vi "Jeffress_model_v009.vi"() -> ()   [LabVIEW 2019]
panel:
  out "element 2":dbl
  out "Elapsed time 2":dbl caption="Get Start Time (s)"
  out "new picture":picture
  out "Left - Right":dbl
  out "Elapsed time 1":dbl caption="Get Start Time (s)"
  in  "stop":bool
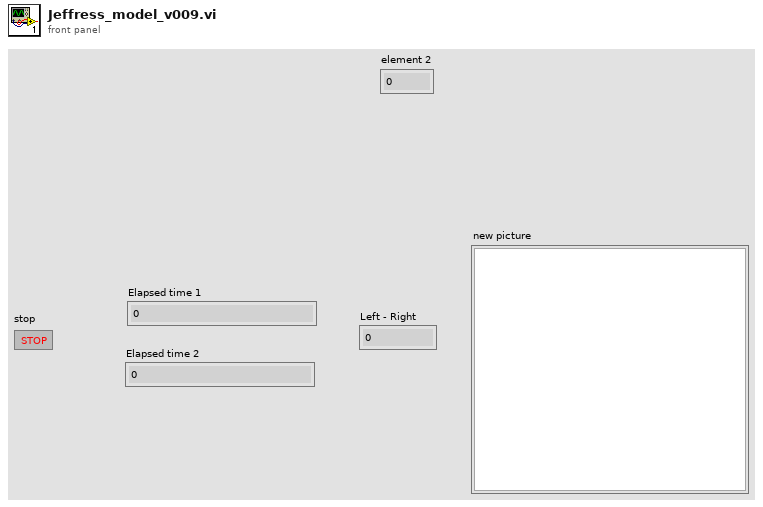
[diagram p1: front panel]
types:
  T1 = cluster{"maximum":dbl, "minimum":dbl, "clip to min":bool, "log?(F)":bool, "grid color":u32, "plot color":u32, "fmt and prec":cluster{"format":enum8{"Decimal", "Scientific", "Engineering", "Binary", "Octal", "Hex"}, "precision":u8}, "visible section":u16}
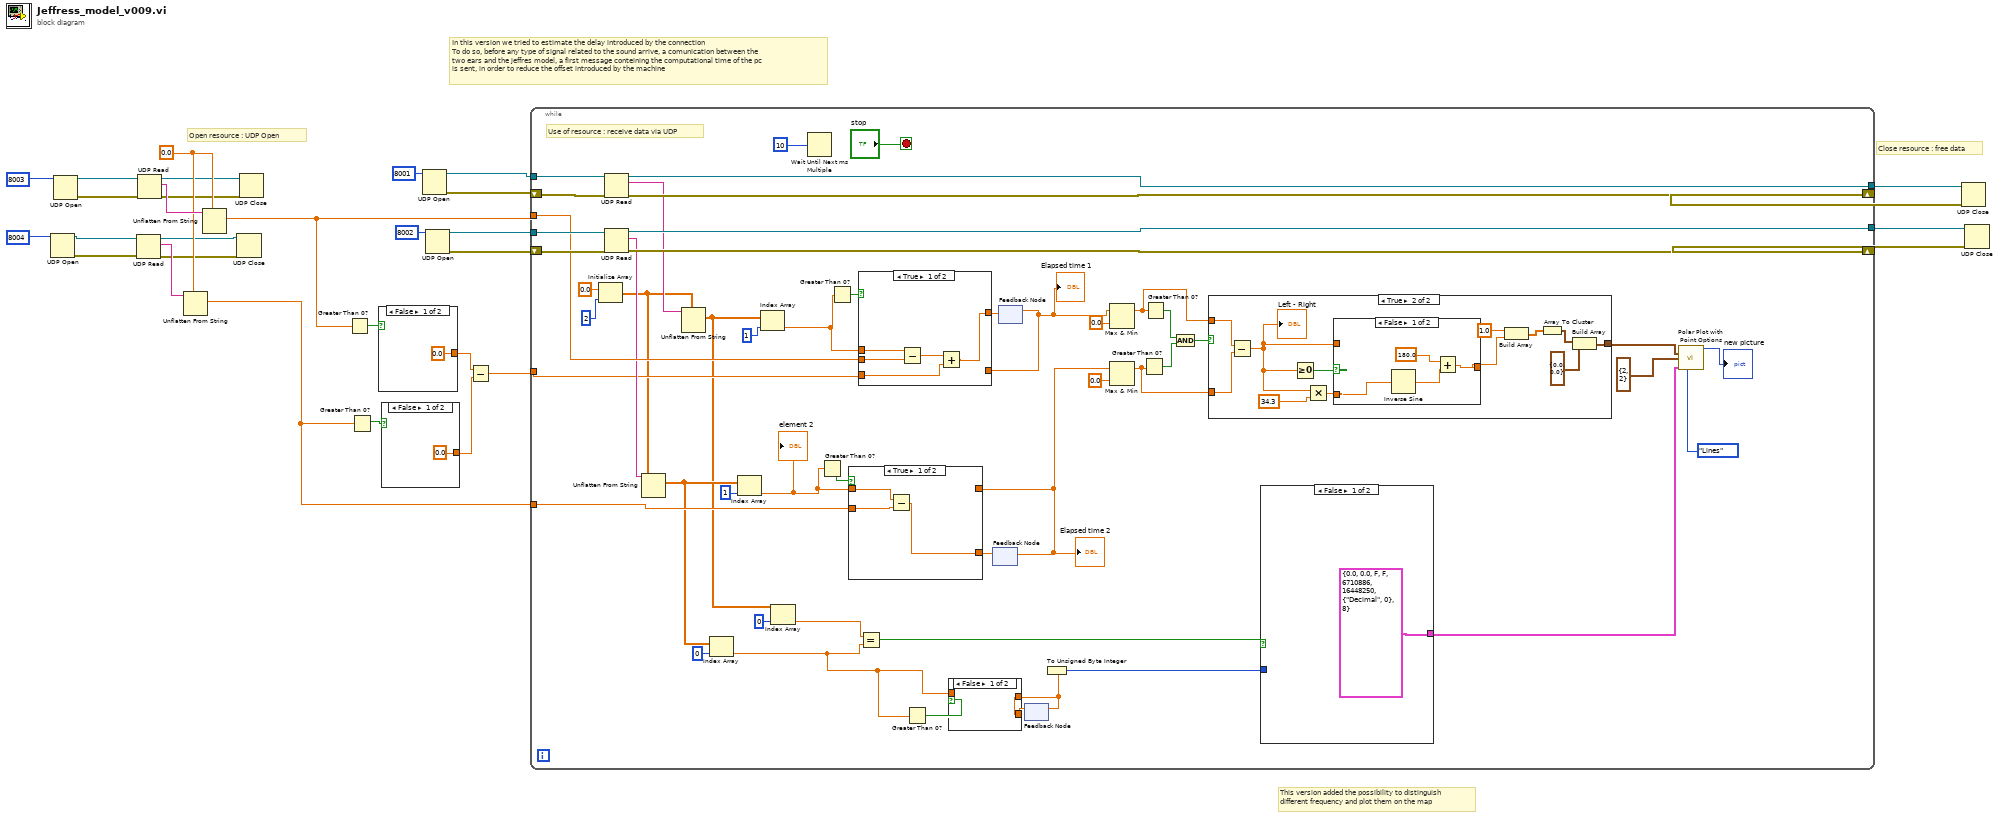
[diagram p0: block diagram]
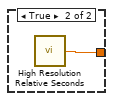
[diagram p2: hidden frame]
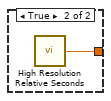
[diagram p3: hidden frame]
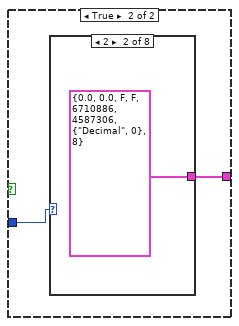
[diagram p5: hidden frame]
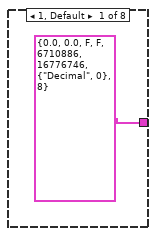
[diagram p6: hidden frame]
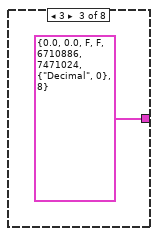
[diagram p7: hidden frame]
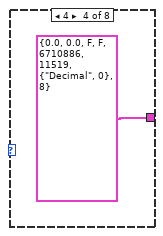
[diagram p8: hidden frame]
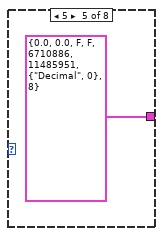
[diagram p9: hidden frame]
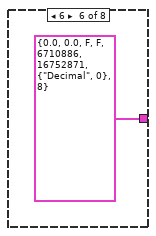
[diagram p10: hidden frame]
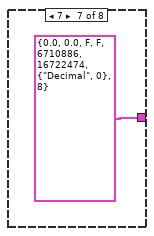
[diagram p11: hidden frame]
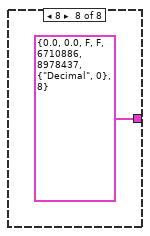
[diagram p12: hidden frame]
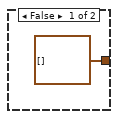
[diagram p14: hidden frame]
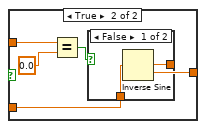
[diagram p15: hidden frame]
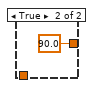
[diagram p16: hidden frame]
diagram:
  w18 = 0.0
  # "This version added the possibility to distinguish\ndifferent frequency and plot them on the map"
  # "In this version we tried to estimate the delay introduced by the connection\nTo do so, before any type of signal related to the sound arrive, a comunication between the\ntwo ears and the jeffres model, a first message conteining the computational time of the pc\nis sent, in order to reduce the offset introduced by the machine"
  # "Close resource : free data"
  # "Open resource : UDP Open"
  n1 = UDP Open(11:u16 8004) -> (port=w22:refnum<k16>, 0:w21:errorcluster)  [unwired: 4 in, 1 out]
  n2 = UDP Open(11:u16 8003) -> (port=w24:refnum<k16>, 0:w23:errorcluster)  [unwired: 4 in, 1 out]
  n3 = UDP Read(connection ID=w22, 8:w21) -> (data out=w19:string, error out=w14:errorcluster, 3:w15:refnum<k16>)  [unwired: 2 in, 2 out]
  n4 = UDP Read(connection ID=w24, 8:w23) -> (data out=w20:string, error out=w16:errorcluster, 3:w17:refnum<k16>)  [unwired: 2 in, 2 out]
  n5 = Unflatten From String(type=w18, binary string=w19) -> (value=w4:dbl)  [unwired: 3 in, 2 out]
  n6 = Unflatten From String(type=w18, binary string=w20) -> (value=w6:dbl)  [unwired: 3 in, 2 out]
  n7 = UDP Close(connection ID=w15, 8:w14) -> ()  [unwired: 2 out]
  n8 = UDP Close(connection ID=w17, 8:w16) -> ()  [unwired: 2 out]
  n9 = Greater Than 0?(x=w6) -> (x > 0?=w7:bool)
  n10 = Greater Than 0?(x=w4) -> (x > 0?=w5:bool)
  n11 = case shown="False" w7 {
    tunnel: [0.0 ("relative seconds") w32] -> w3
    frame False {
    }
    frame True {
      n12 = call <vilib>:"High Resolution Relative Seconds.vi"() -> ("relative seconds"=w32:dbl)
    }
  }
  n13 = case shown="False" w5 {
    tunnel: [0.0 ("relative seconds") w34] -> w2
    frame False {
    }
    frame True {
      n14 = call <vilib>:"High Resolution Relative Seconds.vi"() -> ("relative seconds"=w34:dbl)
    }
  }
  n15 = UDP Open(11:u16 8001 ("port")) -> (port=w13:refnum<k16>, 0:w12:errorcluster)  [unwired: 4 in, 1 out]
  n16 = UDP Open(11:u16 8002 ("port")) -> (port=w11:refnum<k16>, 0:w10:errorcluster)  [unwired: 4 in, 1 out]
  n17 = Subtract(x=w3, y=w2) -> (x-y=w1:dbl)
  n18 = while {
    tunnel: w13 -> [w81]
    tunnel: [w80] -> w29
    shift-right: [w83] -> w30
    shift-left: w12 -> [w82]
    tunnel: w11 -> [w69]
    tunnel: [w67] -> w25
    shift-right: [w68] -> w26
    shift-left: w10 -> [w66]
    tunnel: w4 -> [w59]
    tunnel: w6 -> [w58]
    tunnel: w1 -> [w54]
    stop <- "stop" stop-if-true
    # "Use of resource : receive data via UDP"
    n19 = Initialize Array(0.0 ("element"), 2 ("dimension size")) -> (w51:dbl[])
    n20 = UDP Read(connection ID=w81, 8:w82) -> (data out=w61:string, error out=w83:errorcluster, 3:w80:refnum<k16>)  [unwired: 2 in, 2 out]
    n21 = UDP Read(connection ID=w69, 8:w66) -> (data out=w56:string, error out=w68:errorcluster, 3:w67:refnum<k16>)  [unwired: 2 in, 2 out]
    n22 = Unflatten From String(type=w51, binary string=w56) -> (value=w47:dbl[])  [unwired: 3 in, 2 out]
    n23 = Unflatten From String(type=w51, binary string=w61) -> (value=w46:dbl[])  [unwired: 3 in, 2 out]
    n24 = Index Array(array=w47, index=0) -> (element=w37:dbl)
    n25 = Index Array(array=w47, index=1) -> (element=w41:dbl)
    "element 2" <- w41
    n26 = Index Array(array=w46, index=1) -> (element=w49:dbl)
    n27 = Index Array(array=w46, index=0) -> (element=w43:dbl)
    n28 = Wait Until Next ms Multiple(millisecond multiple=u32 10) -> ()  [unwired: 1 out]
    n29 = Greater Than 0?(x=w41) -> (x > 0?=w55:bool)
    n30 = Greater Than 0?(x=w49) -> (x > 0?=w60:bool)
    n31 = Equal?(x=w43, y=w37) -> (x = y?=w42:bool)
    n32 = Greater Than 0?(x=w37) -> (x > 0?=w38:bool)
    n33 = feedback #1() -> (w57:dbl)  [unwired: 1 in]
    "Elapsed time 2" <- w57
    n34 = case shown="True" w55 {
      tunnel: [w130 w133] -> w64
      tunnel: w57 -> [_ w133]
      tunnel: w41 -> [w132 _]
      tunnel: w59 -> [w131 _]
      frame True {
        n35 = Subtract(x=w132, y=w131) -> (x-y=w130:dbl)
      }
      frame False, Default {
      }
    }
    n36 = feedback-in #1(w64) -> ()
    n37 = feedback #2() -> (w62:dbl)  [unwired: 1 in]
    "Elapsed time 1" <- w62
    n38 = case shown="True" w60 {
      tunnel: [w100 w104] -> w63
      tunnel: w62 -> [_ w104]
      tunnel: w58 -> [w103 _]
      tunnel: w49 -> [w102 _]
      tunnel: w54 -> [w99 _]
      frame True {
        n39 = Subtract(x=w102, y=w103) -> (x-y=w101:dbl)
        n40 = Add(x=w101, y=w99) -> (x+y=w100:dbl)
      }
      frame False {
      }
    }
    n41 = feedback-in #2(w63) -> ()
    n42 = feedback #3() -> (w35:dbl)  [unwired: 1 in]
    n43 = case shown="False" w38 {
      tunnel: w37 -> [_ w87]
      tunnel: [w86 w87] -> w36
      tunnel: w35 -> [w86 _]
      frame False {
      }
      frame True {
      }
    }
    n44 = feedback-in #3(w36) -> ()
    n45 = To Unsigned Byte Integer(number=w35) -> (unsigned 8bit integer=w39:u8)
    n46 = Max & Min(x=w62, y=0.0) -> (max(x,y)=w74:dbl)  [unwired: 1 out]
    n47 = Max & Min(x=w57, y=0.0) -> (max(x,y)=w75:dbl)  [unwired: 1 out]
    n48 = Greater Than 0?(x=w75) -> (x > 0?=w76:bool)
    n49 = Greater Than 0?(x=w74) -> (x > 0?=w77:bool)
    n50 = And(x=w77, y=w76) -> (x .and. y?=w65:bool)
    n51 = case shown="True" w65 {
      tunnel: w74 -> [_ w116]
      tunnel: w75 -> [_ w117]
      tunnel: [cluster{"[0]":dbl, "[1]":dbl}[] [] w111] -> w73
      frame False {
      }
      frame True {
        n52 = Subtract(x=w116, y=w117) -> (x-y=w106:dbl)
        "Left - Right" <- w106
        n53 = Greater Or Equal To 0?(x=w106) -> (x >= 0?=w115:bool)
        n54 = Multiply(x=w106, y=34.3) -> (x*y=w110:dbl)
        n55 = case shown="False" w115 {
          tunnel: w110 -> [w121 w125]
          tunnel: [w120 w126] -> w109
          tunnel: w106 -> [_ w122]
          frame False {
            n56 = Inverse Sine(1:w121) -> (0:w119:dbl)
            n57 = Add(x=180.0, y=w119) -> (x+y=w120:dbl)
          }
          frame True {
            n58 = Equal?(x=w122, y=0.0 ("x")) -> (x = y?=w124:bool)
            n59 = case shown="False" w124 {
              tunnel: [w128 90.0] -> w126
              tunnel: w125 -> [w127 _]
              frame False {
                n60 = Inverse Sine(1:w127) -> (0:w128:dbl)
              }
              frame True {
              }
            }
          }
        }
        n61 = Build Array(1.0 ("element"), w109) -> (w113:dbl[])
        n62 = Array To Cluster(array=w113) -> (cluster=w112:cluster{"[0]":dbl, "[1]":dbl})
        n63 = Build Array(w112, cluster{"[0]":dbl, "[1]":dbl} {"[0]"=0.0, "[1]"=0.0} ("element")) -> (w111:cluster{"[0]":dbl, "[1]":dbl}[])
      }
    }
    n64 = case shown="False" w42 {
      tunnel: w39 -> [_ w90]
      tunnel: [T1 {"maximum"=0.0, "minimum"=0.0, "clip to min"=FALSE, "log?(F)"=FALSE, "grid color"=6710886, "plot color"=16448250, "fmt and prec"={"format"=enum."Decimal", "precision"=0}, "visible section"=8} ("polar attributes") w89] -> w40
      frame False {
      }
      frame True {
        n65 = case shown="2" w90 {
          tunnel: [T1 {"maximum"=0.0, "minimum"=0.0, "clip to min"=FALSE, "log?(F)"=FALSE, "grid color"=6710886, "plot color"=16776746, "fmt and prec"={"format"=enum."Decimal", "precision"=0}, "visible section"=8} ("polar attributes") T1 {"maximum"=0.0, "minimum"=0.0, "clip to min"=FALSE, "log?(F)"=FALSE, "grid color"=6710886, "plot color"=4587306, "fmt and prec"={"format"=enum."Decimal", "precision"=0}, "visible section"=8} ("polar attributes") T1 {"maximum"=0.0, "minimum"=0.0, "clip to min"=FALSE, "log?(F)"=FALSE, "grid color"=6710886, "plot color"=7471024, "fmt and prec"={"format"=enum."Decimal", "precision"=0}, "visible section"=8} ("polar attributes") T1 {"maximum"=0.0, "minimum"=0.0, "clip to min"=FALSE, "log?(F)"=FALSE, "grid color"=6710886, "plot color"=11519, "fmt and prec"={"format"=enum."Decimal", "precision"=0}, "visible section"=8} ("polar attributes") T1 {"maximum"=0.0, "minimum"=0.0, "clip to min"=FALSE, "log?(F)"=FALSE, "grid color"=6710886, "plot color"=11485951, "fmt and prec"={"format"=enum."Decimal", "precision"=0}, "visible section"=8} ("polar attributes") T1 {"maximum"=0.0, "minimum"=0.0, "clip to min"=FALSE, "log?(F)"=FALSE, "grid color"=6710886, "plot color"=16752871, "fmt and prec"={"format"=enum."Decimal", "precision"=0}, "visible section"=8} ("polar attributes") T1 {"maximum"=0.0, "minimum"=0.0, "clip to min"=FALSE, "log?(F)"=FALSE, "grid color"=6710886, "plot color"=16722474, "fmt and prec"={"format"=enum."Decimal", "precision"=0}, "visible section"=8} ("polar attributes") T1 {"maximum"=0.0, "minimum"=0.0, "clip to min"=FALSE, "log?(F)"=FALSE, "grid color"=6710886, "plot color"=8978437, "fmt and prec"={"format"=enum."Decimal", "precision"=0}, "visible section"=8} ("polar attributes")] -> w89
          frame 1, Default {
          }
          frame 2 {
          }
          frame 3 {
          }
          frame 4 {
          }
          frame 5 {
          }
          frame 6 {
          }
          frame 7 {
          }
          frame 8 {
          }
        }
      }
    }
    n66 = call <vilib>:"Polar Plot with Point Options.vi"("data array [mag, phase (deg)]"=w73, "top left point(0, 0)"=cluster{"x":i16, "y":i16} {"x"=2, "y"=2}, "polar attributes"=w40, "Lines/Points"=enum16{"Lines", "Points"}."Lines") -> ("new picture"=→"new picture":picture)  [unwired: 11 in]
  }
  n67 = UDP Close(connection ID=w29, 8:w30) -> ()  [unwired: 2 out]
  n68 = UDP Close(connection ID=w25, 8:w26) -> ()  [unwired: 2 out]
